vi "Flush File Buffers.vi"(8 "error in (no error)":errorcluster, 10 "dwFlags":u32, 11 "BLF File In":refnum<class "Read Write BLF.lvclass">) -> (0 "error out":errorcluster, 3 "BLF File Out":refnum<class "Read Write BLF.lvclass">)   [LabVIEW 2015, in "Read Write BLF.lvclass"]
doc: "This VI will flush a BLF file.\n\n-------------\nBrian Hoover (Hooovahh)"
uses:
  Read Write BLF.lvclass
  Read Write BLF.lvclass/Read Write BLF.ctl
  <vilib>/Utility/error.llb/Error Cluster From Error Code.vi
  <vilib>/Utility/libraryn.llb/Check if File or Folder Exists.vi
  <vilib>/Utility/file.llb/Application Directory.vi
  <vilib>/ErrorRing/Error Ring.xnode
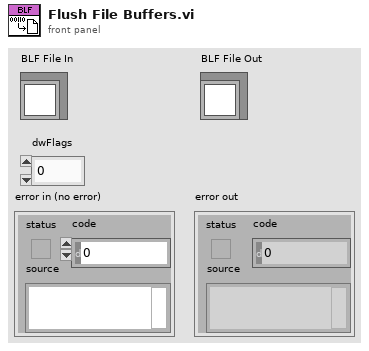
[diagram p1: front panel]
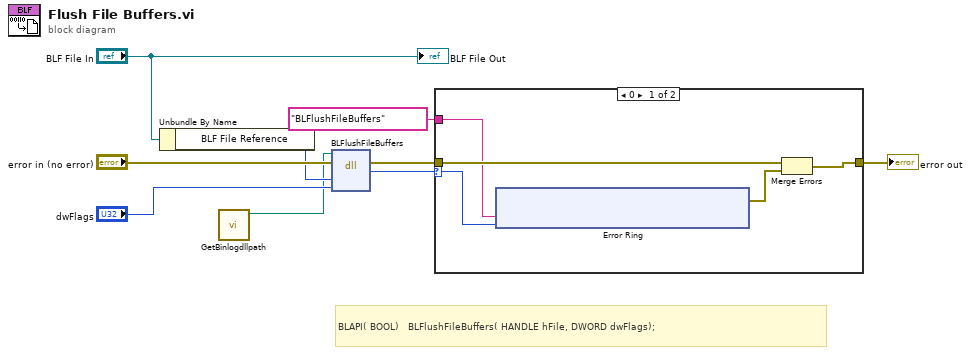
[diagram p0: block diagram]
diagram:
  # "BLAPI( BOOL)   BLFlushFileBuffers( HANDLE hFile, DWORD dwFlags);"
  n1 = Unbundle By Name("BLF File In") -> ("BLF File Reference"=w2:u32)
  n2 = call "GetBinlogdllpath.vi"() -> ("dup path"=w1:path)  [unwired: 11 in]
  n3 = dll-call lib="PTH2Tabs E自开发软件X-CAN项目X-CAN离线分析平台 V2.3.1BLFbinlog.*" fn="BLFlushFileBuffers"(path in=w1, error in="error in (no error)", "hFile"=w2, "dwFlags"="dwFlags") -> (error out=w6:errorcluster, "返回类型"=w5:i32)  [unwired: 3 in, 1 out]
  n4 = case shown="0" w5 {
    selector: w5 -> [w12 _]
    tunnel: w6 -> [w14 w23]
    tunnel: [w13 w23] -> w4
    tunnel: "BLFlushFileBuffers" -> [w11 _]
    frame 0 {
      n5 = xnode "Error Ring"("参数 0"=w11, "参数 1"=w12) -> ("错误输出"=w10:errorcluster)
      n6 = Merge Errors(w14, w10) -> (w13:errorcluster)
    }
    frame Default {
    }
  }
  "error out" <- w4
  "BLF File Out" <- "BLF File In"
